vi "Export All Mappings.vi"(8 "error in (no error)":errorcluster, 11 "Scaling configuration in":refnum<class "Scaling configuration.lvclass">) -> (0 "error out":errorcluster, 2 "mapping sets":T1(array[cluster]), 3 "Scaling configuration out":refnum<class "Scaling configuration.lvclass">)   [LabVIEW 2013, in "Scaling configuration.lvclass"]
uses:
  Scaling configuration.lvclass
  <vilib>/NI/Tag Bus Module Framework/channel/TBM channel.lvclass
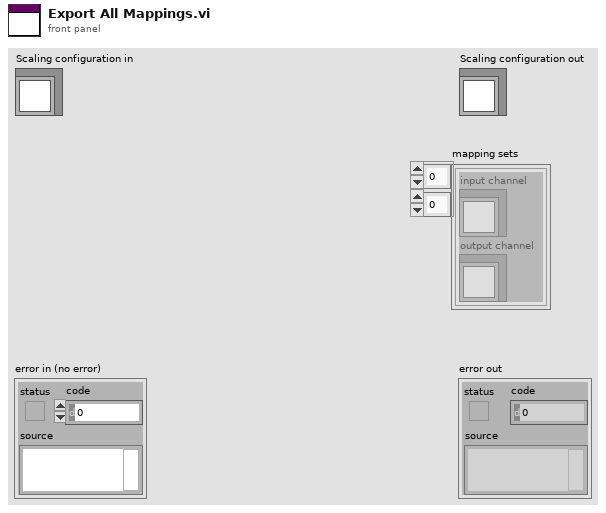
[diagram p1: front panel]
types:
  T1 = cluster{"input channel":refnum<class "TBM channel.lvclass">, "output channel":refnum<class "TBM channel.lvclass">}[][]
  T2 = cluster{"input channel":refnum<class "TBM channel.lvclass">, "output channel":refnum<class "TBM channel.lvclass">}
  T3 = typedef "Scaling configuration.lvclass/scale data types.ctl" = enum16{"Double", "Single", "I64", "I32", "I16", "I8", "U64", "U32", "U16", "U8"}
  T4 = cluster{"mappings":cluster{"input channel":refnum<class "TBM channel.lvclass">, "output channel":refnum<class "TBM channel.lvclass">, "input data type":T3, "output data type":T3}[], "name":string}[]
  T5 = cluster{"input channel":refnum<class "TBM channel.lvclass">, "output channel":refnum<class "TBM channel.lvclass">, "input data type":T3, "output data type":T3}[]
  T6 = cluster{"input channel":refnum<class "TBM channel.lvclass">, "output channel":refnum<class "TBM channel.lvclass">, "input data type":T3, "output data type":T3}
  T7 = cluster{"mappings":cluster{"input channel":refnum<class "TBM channel.lvclass">, "output channel":refnum<class "TBM channel.lvclass">, "input data type":T3, "output data type":T3}[], "name":string}
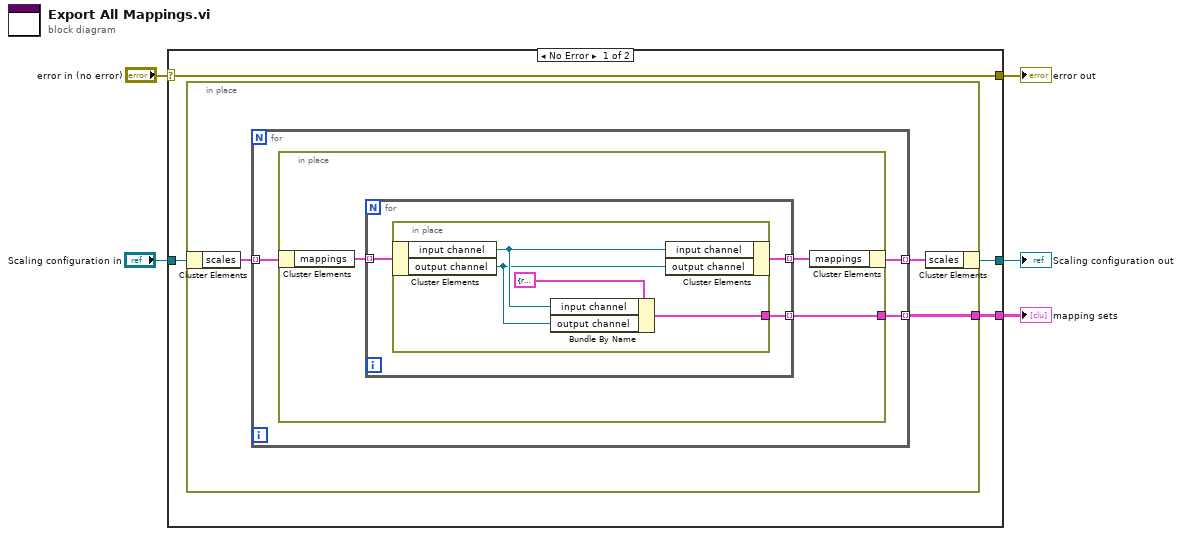
[diagram p0: block diagram]
diagram:
  n1 = case shown="No Error" "error in (no error)" {
    selector: "error in (no error)" -> [w9 w27]
    tunnel: [w9 w27] -> w4
    tunnel: [w7 w26] -> w2
    tunnel: "Scaling configuration in" -> [w8 w26]
    tunnel: [w6 _] -> w1
    frame No Error {
      n2 = in-place {
        in-place-border: [w10] -> w6
        n3 = in-place-cluster #1(w8) -> ("scales"=w12:T4)
        n4 = for {
          tunnel: w12 -> [w15] mode=indexing
          tunnel: [w14] -> w11 mode=indexing
          tunnel: [w13] -> w10 mode=indexing
          n5 = in-place {
            in-place-border: [w16] -> w13
            n6 = in-place-cluster #2(w15) -> ("mappings"=w18:T5)
            n7 = for {
              tunnel: w18 -> [w21] mode=indexing
              tunnel: [w20] -> w17 mode=indexing
              tunnel: [w19] -> w16 mode=indexing
              n8 = in-place {
                in-place-border: [w22] -> w19
                n9 = in-place-cluster #3(w21) -> ("input channel"=w24:refnum<class "TBM channel.lvclass">, "output channel"=w23:refnum<class "TBM channel.lvclass">)
                n10 = Bundle By Name(cluster=T2 {"input channel"=refnum, "output channel"=refnum} ("mapping"), "input channel"=w24, "output channel"=w23) -> (w22:T2)
                n11 = in-place-cluster #3("input channel"=w24, "output channel"=w23) -> (w20:T6)
              }
            }
            n12 = in-place-cluster #2("mappings"=w17) -> (w14:T7)
          }
        }
        n13 = in-place-cluster #1("scales"=w11) -> (w7:refnum<class "Scaling configuration.lvclass">)
      }
    }
    frame Error {
    }
  }
  "error out" <- w4
  "Scaling configuration out" <- w2
  "mapping sets" <- w1
